vi "ex03_front_panel.vi"() -> ()   [LabVIEW 2019]
panel:
  out "LED 4":bool
  in  "SW 4":bool
  in  "SW 3":bool
  out "LED 3":bool
  in  "SW 2":bool
  out "LED 2":bool
  in  "SW":bool
  out "LED":bool
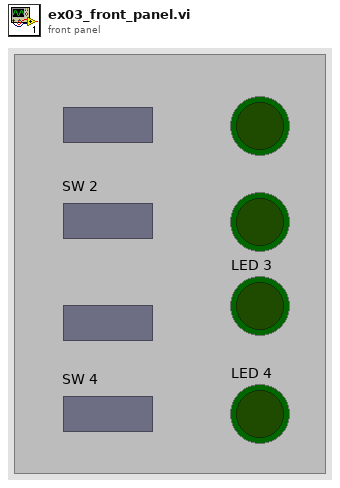
[diagram p1: front panel]
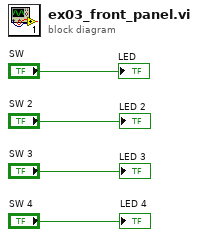
[diagram p0: block diagram]
diagram:
  "LED" <- "SW"
  "LED 2" <- "SW 2"
  "LED 3" <- "SW 3"
  "LED 4" <- "SW 4"
